vi "Set-acceleration.vi"(8 "error in (no error)":errorcluster, 10 "Acceleration":dbl caption="Acceleration [rpm/s]", 11 "Motor in":refnum<class "Motor.lvclass">) -> (0 "error out":errorcluster, 3 "Motor out":refnum<class "Motor.lvclass">)   [LabVIEW 2013, in "PowderDeposition.lvlib" / "Motor.lvclass"]
uses:
  Motor.lvclass
  Motor.lvclass/Motor.ctl
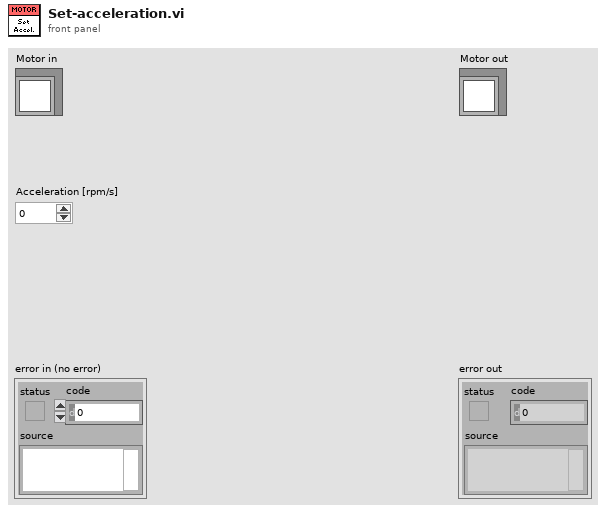
[diagram p1: front panel]
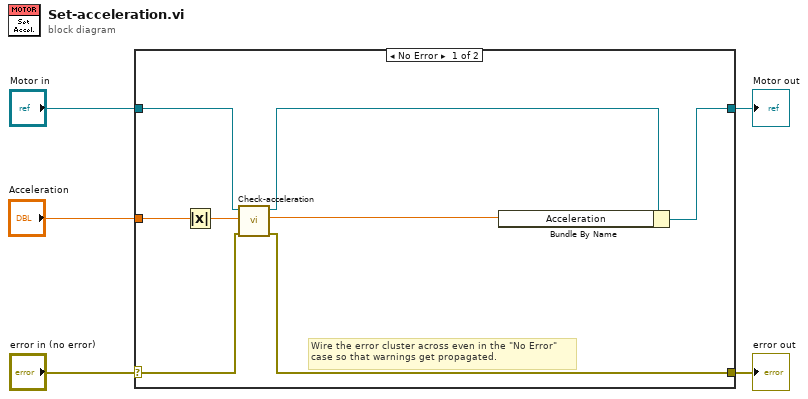
[diagram p0: block diagram]
diagram:
  n1 = case shown="No Error" "error in (no error)" {
    selector: "error in (no error)" -> [w8 w15]
    tunnel: [w7 w15] -> w4
    tunnel: [w13 w14] -> w2
    tunnel: "Motor in" -> [w10 w14]
    tunnel: "Acceleration" -> [w12 _]
    frame No Error {
      # "Wire the error cluster across even in the \"No Error\"\ncase so that warnings get propagated."
      n2 = Absolute Value(x=w12) -> (abs(x)=w11:dbl)
      n3 = call-dynamic "Check-acceleration.vi"("error in (no error)"=w8, "Acceleration in"=w11, "Motor in"=w10) -> ("error out"=w7:errorcluster, "Acceleration out"=w6:dbl, "Motor out"=w9:refnum<class "Motor.lvclass">)  [unwired: 5 in, 1 out]
      n4 = Bundle By Name(cluster=w9, "Acceleration"=w6) -> (w13:refnum<class "Motor.lvclass">)
    }
    frame Error {
    }
  }
  "error out" <- w4
  "Motor out" <- w2
